vi "RealTime_main.vi"() -> ()   [LabVIEW 2020]
uses:
  <vilib>/rvi/interface/nirviOpenFPGA/nirviOpenFPGA.xnode
  <vilib>/rvi/interface/nirviReadWriteControl/nirviReadWriteControl.xnode
  NiFpgaLv.dll
  <vilib>/Utility/error.llb/Error Cluster From Error Code.vi
  <vilib>/rvi/interface/Simulation/niFpgaSimulationCallBeginRW.vi
  <vilib>/rvi/errors/niLvFpgaAdjustHostInterfaceError.vi
  <vilib>/rvi/interface/nirviMethod/nirviMethod.xnode
  <vilib>/rvi/errors/niLvFpgaMergeErrorWithErrorCode.vi
  <vilib>/FPGAPlugInAG/Dynamic/niLvFpga_Run_Dynamic.vi
  <vilib>/platform/TimedLoop/XDataNode/XDataNode.xnode
  <vilib>/Platform/TimedLoop/XDataNode/nitl_modes.ctl
  <vilib>/Platform/TimedLoop/XDataNode/XDNodeRunTimeDep.lvlib
  <vilib>/Platform/TimedLoop/XDataNode/wakeup.ctl
  <vilib>/Platform/TimedLoop/XDataNode/timing_clust.ctl
  <vilib>/rvi/interface/nirviCloseFPGA/nirviCloseFPGA.xnode
  <vilib>/FPGAPlugInAG/Dynamic/niLvFpga_ReadFifo_Dynamic.vi
  <vilib>/FPGAPlugInAG/Dynamic/niLvFpga_ConfigureFifo_Dynamic.vi
  <vilib>/FPGAPlugInAG/Dynamic/niLvFpga_StartFifo_Dynamic.vi
  <vilib>/FPGAPlugInAG/Dynamic/niLvFpga_Close_Dynamic.vi
  FPGA Bitfiles/datalogger_FPGATarget_FPGAmain_74o0pMjR1D4.lvbitx
  FPGA_main.vi
  <vilib>/FPGAPlugInAG/myRIO-1900/niLvFpga_Open_myRIO-1900.vi
  <vilib>/rvi/interface/common/dynamic/niFpgaDynamicAddResources.vi
panel:
  out "Waveform Graph":i16[][](graph)
  in  "Monitoring?":bool
  in  "SamplesOverThreshold (<255)":u8
  in  "TriggerZ":i16(slide) scale=0.0..500.0
  in  "TriggerY":i16(slide) scale=0.0..500.0
  in  "TriggerX":i16(slide) scale=0.0..500.0
  in  "stop":bool
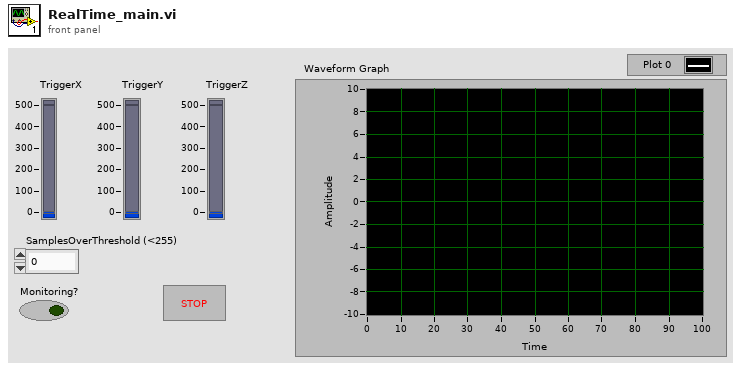
[diagram p1: front panel]
types:
  T1 = typedef "XDNodeRunTimeDep.lvlib/timing_clust.ctl" = cluster{"Expected End [f-1]":u64, "Actual End [f-1]":u64, "Finished Late? [f-1]":bool, "Expected End [i-1]":u64, "Actual End [i-1]":u64, "Finished Late? [i-1]":bool, "Expected Start [i]":u64, "Actual Start [i]":u64, "Expected Start [f]":u64, "Actual Start [f]":u64, "Source Name":string, "Structure Name":string, "Period":i64, "Deadline":i64, "Offset":i64, "Start":i64, "Priority":i32, "Timeout":i32, "Mode":T2, "Wakeup Reason":T3, "Error":errorcluster, "Source Type":string, "Secondary Source Type":string, "Global End Time":u64, "Global Start Time":u64, "Frame Duration":u64, "Iteration Duration":u64, "Assigned CPU":i32, "I/O Scan Engine Mode":u32}
  T2 = typedef "XDNodeRunTimeDep.lvlib/nitl_modes.ctl" = enum32{"No Change", "Process missed periods, maintain original phase", "Discard missed periods, maintain original phase", "Process missed periods, ignore original phase", "Discard missed periods, ignore original phase"}
  T3 = typedef "XDNodeRunTimeDep.lvlib/wakeup.ctl" = enum32{"Normal", "Aborted", "Asynchronous wakeup", "Timing source error", "Timed loop error", "Timeout"}
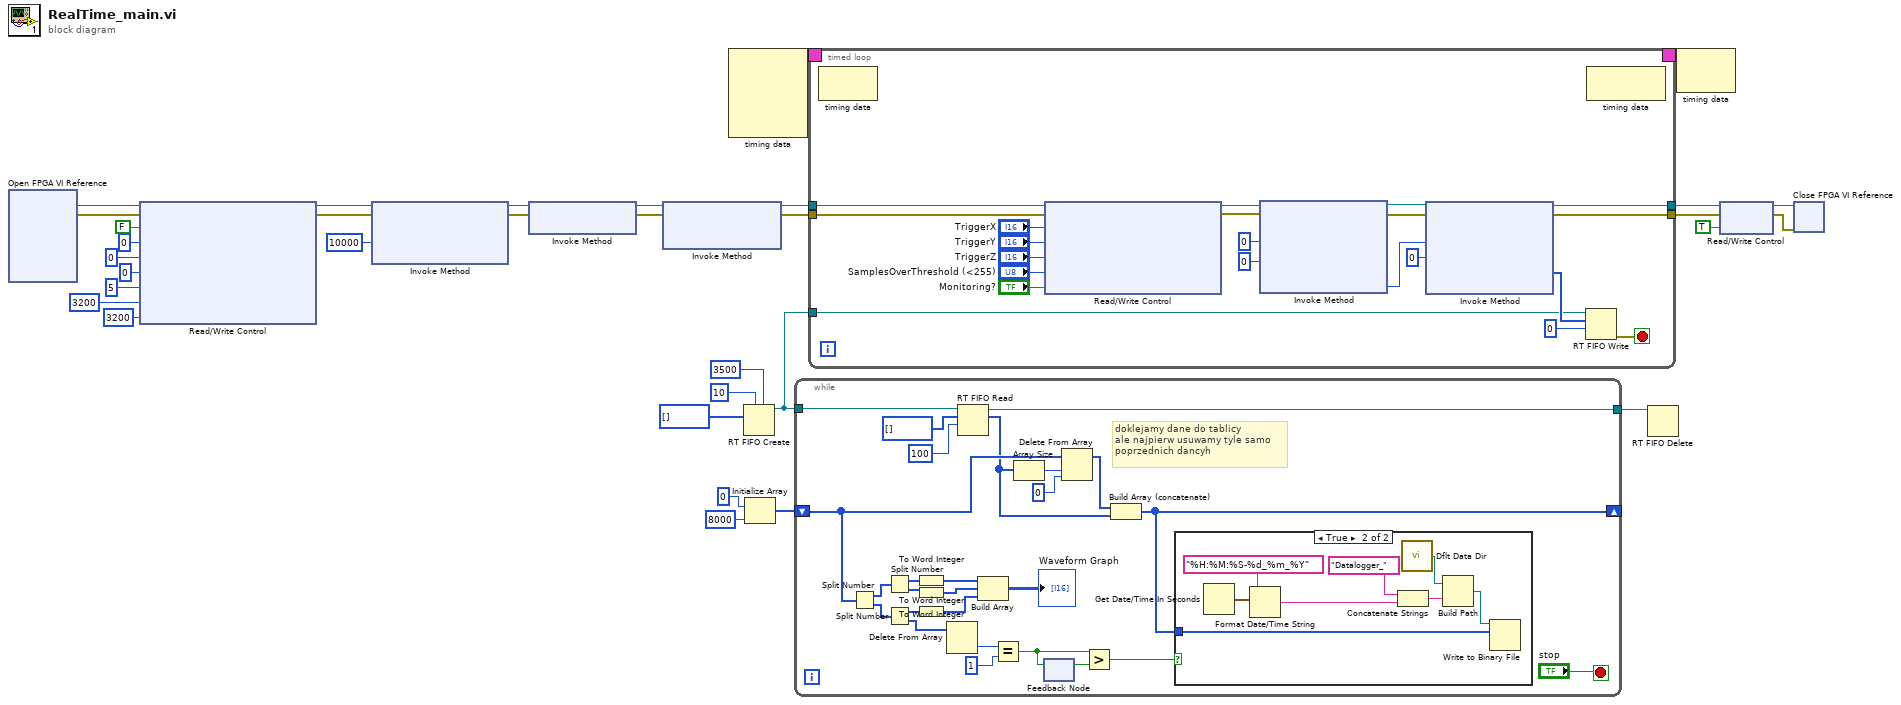
[diagram p0: block diagram]
diagram:
  n1 = xnode "Open FPGA VI Reference"() -> ("FPGA VI Reference Out"=w33:refnum<k20>, "error out"=w23:errorcluster)  [unwired: 2 in]
  n2 = xnode "Read/Write Control"("FPGA VI Reference In"=w33, "error in"=w23, "stop"=FALSE, "TriggerX"=i16 0, "TriggerY"=i16 0, "TriggerZ"=i16 0, "SamplesOverThreshold (<255)"=u8 5 ("SamplesOverThreshold"), "PreTriggerDataLength"=u16 3200, "PostTriggerDataLength"=u16 3200) -> ("FPGA VI Reference Out"=w28:refnum<k20>, "error out"=w22:errorcluster)
  n3 = xnode "Invoke Method"("FPGA VI Reference In"=w28, "error in"=w22, "Requested Depth"=u32 10000) -> ("FPGA VI Reference Out"=w26:refnum<k20>, "error out"=w21:errorcluster)  [unwired: 1 out]
  n4 = xnode "Invoke Method"("FPGA VI Reference In"=w26, "error in"=w21) -> ("FPGA VI Reference Out"=w25:refnum<k20>, "error out"=w24:errorcluster)
  n5 = xnode "Invoke Method"("FPGA VI Reference In"=w25, "error in"=w24) -> ("FPGA VI Reference Out"=w20:refnum<k20>, "error out"=w19:errorcluster)  [unwired: 1 in]
  n6 = node-c288() -> (w18:T1)  [unwired: 4 in]
  n7 = RT FIFO Create(1:u64[] [] ("Data"), 4:u32 10 ("size (10)"), 6:u32 3500 ("elements in array (1)")) -> (8:w5:refnum<k33>)  [unwired: 5 in, 2 out]
  n8 = Initialize Array(u64 0 ("element"), 8000 ("dimension size")) -> (w4:u64[])
  n9 = while {
    tunnel: w5 -> [w58]
    shift-right: [w37] -> _
    shift-left: w4 -> [w42]
    tunnel: [w52] -> w1
    stop <- "stop" stop-if-true
    # "doklejamy dane do tablicy\nale najpierw usuwamy tyle samo\npoprzednich dancyh"
    n10 = Split Number(x=w42) -> (hi(x)=w51:u32[], lo(x)=w50:u32[])
    n11 = Split Number(x=w51) -> (hi(x)=w49:u16[], lo(x)=w48:u16[])
    n12 = Split Number(x=w50) -> (hi(x)=w47:u16[], lo(x)=w40:u16[])
    n13 = To Word Integer(number=w49) -> (16bit integer=w46:i16[])
    n14 = To Word Integer(number=w48) -> (16bit integer=w45:i16[])
    n15 = To Word Integer(number=w47) -> (16bit integer=w44:i16[])
    n16 = Delete From Array(array=w40) -> (deleted portion=w39:u16)  [unwired: 2 in, 1 out]
    n17 = RT FIFO Read(0:w58, 1:u64[] [] ("element"), 2:100 ("timeout in ms (0)")) -> (8:w52:refnum<k33>, 9:w41:u64[])  [unwired: 1 in, 3 out]
    n18 = Build Array(w46, w45, w44) -> (→"Waveform Graph":i16[][])
    n19 = Equal?(x=w39, y=u16 1 ("x")) -> (x = y?=w34:bool)
    n20 = Array Size(array=w41) -> (size(s)=w55:i32)
    n21 = feedback-in #1(w34) -> ()
    n22 = feedback #1() -> (w35:bool)  [unwired: 1 in]
    n23 = Delete From Array(array=w42, length=w55, index=0) -> (array with subset deleted=w53:u64[])  [unwired: 1 out]
    n24 = Greater?(x=w34, y=w35) -> (0:w36:bool)
    n25 = Build Array (concatenate)(w53, w41) -> (w37:u64[])
    n26 = case shown="True" w36 {
      tunnel: w37 -> [_ w67]
      frame False {
      }
      frame True {
        n27 = Get Date/Time In Seconds() -> (seconds since 1Jan1904=w66:timestamp)
        n28 = Format Date/Time String(time format string (%c)="%H:%M:%S-%d_%m_%Y", seconds (now)=w66) -> (date/time string=w64:string)  [unwired: 1 in]
        n29 = Concatenate Strings("Datalogger_" ("string"), w64) -> (w62:string)
        n30 = call <vilib>:"Dflt Data Dir.vi"() -> ("App:Default Data Directory"=w61:path)
        n31 = Build Path(base path=w61, name or relative path=w62) -> (appended path=w60:path)
        n32 = Write to Binary File(file (use dialog)=w60, data=w67) -> ()  [unwired: 4 in, 3 out]
      }
    }
  }
  n33 = timed-loop {
    timing: w18 -> [_]
    timing-out: [_] -> w17
    tunnel: w20 -> [w88]
    tunnel: w19 -> [w87]
    tunnel: [w86] -> w16
    tunnel: [w85] -> w14
    tunnel: w5 -> [w68]
    stop <- w70 stop-if-true
    n34 = node-c288() -> ()  [unwired: 1 in, 1 out]
    n35 = xnode "Read/Write Control"("FPGA VI Reference In"=w88, "error in"=w87, "TriggerX"="TriggerX", "TriggerY"="TriggerY", "TriggerZ"="TriggerZ", "SamplesOverThreshold (<255)"="SamplesOverThreshold (<255)", "Monitoring?"="Monitoring?") -> ("FPGA VI Reference Out"=w80:refnum<k20>, "error out"=w77:errorcluster)
    n36 = xnode "Invoke Method"("FPGA VI Reference In"=w80, "error in"=w77, "Number of Elements"=u32 0, "Timeout (ms)"=0) -> ("FPGA VI Reference Out"=w79:refnum<k20>, "error out"=w78:errorcluster, "Elements Remaining"=w74:u32)  [unwired: 1 out]
    n37 = xnode "Invoke Method"("FPGA VI Reference In"=w79, "error in"=w78, "Number of Elements"=w74, "Timeout (ms)"=0) -> ("FPGA VI Reference Out"=w86:refnum<k20>, "error out"=w85:errorcluster, "Data"=w71:u64[])  [unwired: 1 out]
    n38 = RT FIFO Write(0:w68, 1:w71, 2:0 ("timeout in ms (0)")) -> (11:w70:errorcluster)  [unwired: 2 in, 3 out]
    n39 = node-c288() -> ()  [unwired: 1 in, 1 out]
  }
  n40 = RT FIFO Delete(0:w1) -> ()  [unwired: 2 in, 1 out]
  n41 = node-c288(w17) -> ()  [unwired: 1 out]
  n42 = xnode "Read/Write Control"("FPGA VI Reference In"=w16, "error in"=w14, "stop"=TRUE) -> ("FPGA VI Reference Out"=w13:refnum<k20>, "error out"=w12:errorcluster)
  n43 = xnode "Close FPGA VI Reference"("FPGA VI Reference In"=w13, "error in"=w12) -> ()  [unwired: 1 out]
